vi "DMM Configuration - Disable Temp Controls.vi"(8 "error in (no error)":errorcluster, 11 "Measurement Controls Refs":T1) -> (0 "error out":errorcluster)   [LabVIEW 2016, in "DMM-SWITCH-ScanList System Explorer.lvlib"]
uses:
  DMM-SWITCH-ScanList System Explorer.lvlib
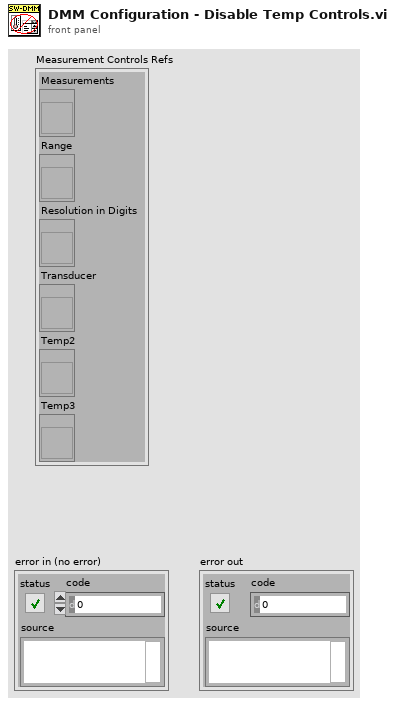
[diagram p1: front panel]
types:
  T1 = cluster{"Measurements":refnum<vi>, "Range":refnum<vi>, "Resolution in Digits":refnum<vi>, "Transducer":refnum<vi>, "Temp2":refnum<vi>, "Temp3":refnum<vi>}
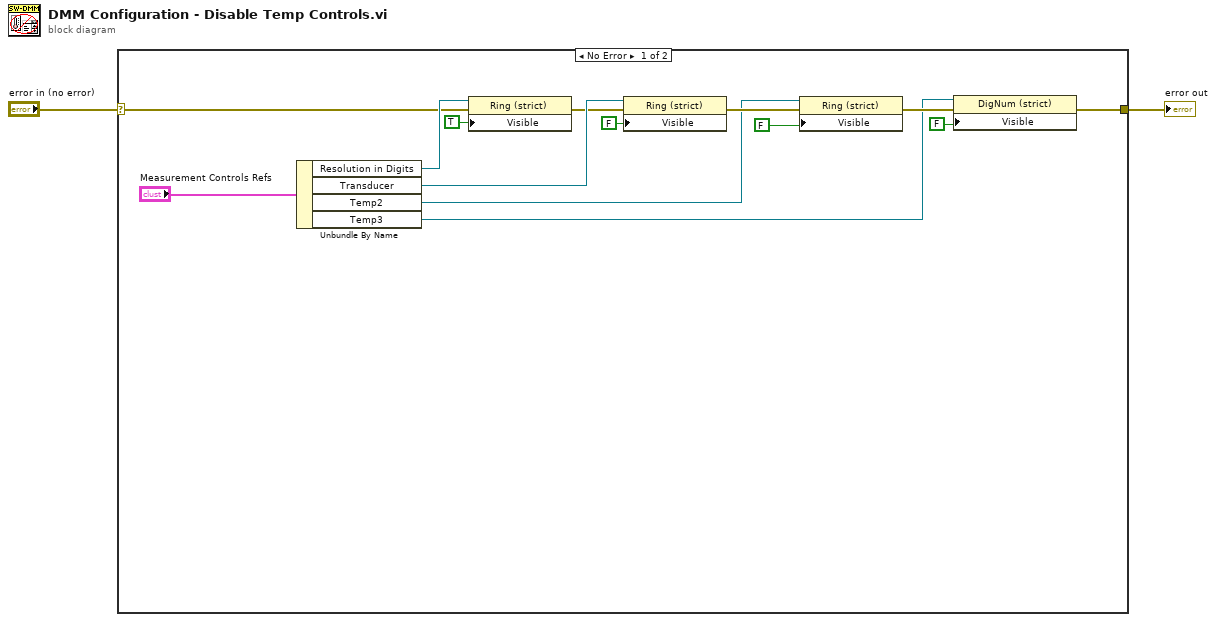
[diagram p0: block diagram]
diagram:
  n1 = case shown="No Error" "error in (no error)" {
    selector: "error in (no error)" -> [w6 w17]
    tunnel: [w14 w17] -> w2
    frame No Error {
      n2 = Unbundle By Name("Measurement Controls Refs") -> ("Resolution in Digits"=w16:refnum<vi>, "Transducer"=w15:refnum<vi>, "Temp2"=w3:refnum<vi>, "Temp3"=w4:refnum<vi>)
      n3 = property on="Property Node" class="Ring (strict)"(reference=w16, error in=w6, "Visible"=TRUE) -> (error out=w11:errorcluster)  [unwired: 1 out]
      n4 = property on="Property Node" class="Ring (strict)"(reference=w15, error in=w11, "Visible"=FALSE) -> (error out=w9:errorcluster)  [unwired: 1 out]
      n5 = property on="Property Node" class="Ring (strict)"(reference=w3, error in=w9, "Visible"=FALSE) -> (error out=w7:errorcluster)  [unwired: 1 out]
      n6 = property on="Property Node" class="DigNum (strict)"(reference=w4, error in=w7, "Visible"=FALSE) -> (error out=w14:errorcluster)  [unwired: 1 out]
    }
    frame Error {
    }
  }
  "error out" <- w2
